vi "Global_ASI_stage.vi"() -> ()   [LabVIEW 2015]
panel:
  out "ASI ready":bool
  out "BF":bool
  out "ASI done":bool
  out "ASI start":bool
  out "XYZ":cluster{"x(um)":dbl, "y(um)":dbl, "z(um)":dbl} {"x(um)" format="%#.1f"; "y(um)" format="%#.1f"; "z(um)" format="%#.1f"}
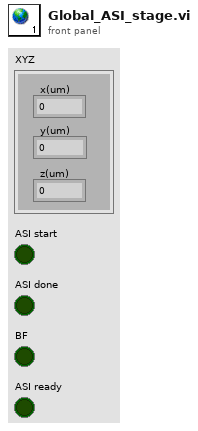
[diagram p1: front panel]
diagram:
